vi "Matlab Chirps Computation.vi"(7 "Movement correction":bool, 8 "error in":errorcluster, 9 "Zoom":dbl[](array[numeric]), 10 "ROI Coordinates":T3={"XYZ Start"=[{"X"=-1.0, "Y"=-1.0, "Z"=0.0}, {"X"=-1.0, "Y"=-0.99, "Z"=0.0}, {"X"=-1.0, "Y"=-0.98, "Z"=0.0}, {"X"=-1.0, "Y"=-0.97, "Z"=0.0}, {"X"=-1.0, "Y"=-0.96, "Z"=0.0}, {"X"=-1.0, "Y"=-0.95, "Z"=0.0}, {"X"=-1.0, "Y"=-0.94, "Z"=0.0}, {"X"=-1.0, "Y"=-0.93, "Z"=0.0}, {"X"=-1.0, "Y"=-0.92, "Z"=0.0}, {"X"=-1.0, "Y"=-0.91, "Z"=0.0}, {"X"=-1.0, "Y"=-0.9, "Z"=0.0}, {"X"=-1.0, "Y"=-0.89, "Z"=0.0}, {"X"=-1.0, "Y"=-0.88, "Z"=0.0}, {"X"=-1.0, "Y"=-0.87, "Z"=0.0}, {"X"=-1.0, "Y"=-0.86, "Z"=0.0}, {"X"=-1.0, "Y"=-0.85, "Z"=0.0}, {"X"=-1.0, "Y"=-0.84, "Z"=0.0}, {"X"=-1.0, "Y"=-0.83, "Z"=0.0}, {"X"=-1.0, "Y"=-0.82, "Z"=0.0}, {"X"=-1.0, "Y"=-0.81, "Z"=0.0}, {"X"=-1.0, "Y"=-0.8, "Z"=0.0}, {"X"=-1.0, "Y"=-0.79, "Z"=0.0}, {"X"=-1.0, "Y"=-0.78, "Z"=0.0}, {"X"=-1.0, "Y"=-0.77, "Z"=0.0}, {"X"=-1.0, "Y"=-0.76, "Z"=0.0}, {"X"=-1.0, "Y"=-0.75, "Z"=0.0}, {"X"=-1.0, "Y"=-0.74, "Z"=0.0}, {"X"=-1.0, "Y"=-0.73, "Z"=0.0}, {"X"=-1.0, "Y"=-0.72, "Z"=0.0}, {"X"=-1.0, "Y"=-0.71, "Z"=0.0}, {"X"=-1.0, "Y"=-0.7, "Z"=0.0}, {"X"=-1.0, "Y"=-0.69, "Z"=0.0}, {"X"=-1.0, "Y"=-0.68, "Z"=0.0}, {"X"=-1.0, "Y"=-0.67, "Z"=0.0}, {"X"=-1.0, "Y"=-0.66, "Z"=0.0}, {"X"=-1.0, "Y"=-0.65, "Z"=0.0}, {"X"=-1.0, "Y"=-0.64, "Z"=0.0}, {"X"=-1.0, "Y"=-0.63, "Z"=0.0}, {"X"=-1.0, "Y"=-0.62, "Z"=0.0}, {"X"=-1.0, "Y"=-0.61, "Z"=0.0}, {"X"=-1.0, "Y"=-0.6, "Z"=0.0}, {"X"=-1.0, "Y"=-0.59, "Z"=0.0}, {"X"=-1.0, "Y"=-0.58, "Z"=0.0}, {"X"=-1.0, "Y"=-0.57, "Z"=0.0}, {"X"=-1.0, "Y"=-0.56, "Z"=0.0}, {"X"=-1.0, "Y"=-0.55, "Z"=0.0}, {"X"=-1.0, "Y"=-0.54, "Z"=0.0}, {"X"=-1.0, "Y"=-0.53, "Z"=0.0}, {"X"=-1.0, "Y"=-0.52, "Z"=0.0}, {"X"=-1.0, "Y"=-0.51, "Z"=0.0}, {"X"=-1.0, "Y"=-0.5, "Z"=0.0}, {"X"=-1.0, "Y"=-0.49, "Z"=0.0}, {"X"=-1.0, "Y"=-0.48, "Z"=0.0}, {"X"=-1.0, "Y"=-0.47, "Z"=0.0}, {"X"=-1.0, "Y"=-0.46, "Z"=0.0}, {"X"=-1.0, "Y"=-0.45, "Z"=0.0}, {"X"=-1.0, "Y"=-0.44, "Z"=0.0}, {"X"=-1.0, "Y"=-0.43, "Z"=0.0}, {"X"=-1.0, "Y"=-0.42, "Z"=0.0}, {"X"=-1.0, "Y"=-0.41, "Z"=0.0}, {"X"=-1.0, "Y"=-0.4, "Z"=0.0}, {"X"=-1.0, "Y"=-0.39, "Z"=0.0}, {"X"=-1.0, "Y"=-0.38, "Z"=0.0}, {"X"=-1.0, "Y"=-0.37, "Z"=0.0}, {"X"=-1.0, "Y"=-0.36, "Z"=0.0}, {"X"=-1.0, "Y"=-0.35, "Z"=0.0}, {"X"=-1.0, "Y"=-0.34, "Z"=0.0}, {"X"=-1.0, "Y"=-0.33, "Z"=0.0}, {"X"=-1.0, "Y"=-0.32, "Z"=0.0}, {"X"=-1.0, "Y"=-0.31, "Z"=0.0}, {"X"=-1.0, "Y"=-0.3, "Z"=0.0}, {"X"=-1.0, "Y"=-0.29, "Z"=0.0}, {"X"=-1.0, "Y"=-0.28, "Z"=0.0}, {"X"=-1.0, "Y"=-0.27, "Z"=0.0}, {"X"=-1.0, "Y"=-0.26, "Z"=0.0}, {"X"=-1.0, "Y"=-0.25, "Z"=0.0}, {"X"=-1.0, "Y"=-0.24, "Z"=0.0}, {"X"=-1.0, "Y"=-0.23, "Z"=0.0}, {"X"=-1.0, "Y"=-0.22, "Z"=0.0}, {"X"=-1.0, "Y"=-0.21, "Z"=0.0}, {"X"=-1.0, "Y"=-0.2, "Z"=0.0}, {"X"=-1.0, "Y"=-0.19, "Z"=0.0}, {"X"=-1.0, "Y"=-0.18, "Z"=0.0}, {"X"=-1.0, "Y"=-0.17, "Z"=0.0}, {"X"=-1.0, "Y"=-0.16, "Z"=0.0}, {"X"=-1.0, "Y"=-0.15, "Z"=0.0}, {"X"=-1.0, "Y"=-0.14, "Z"=0.0}, {"X"=-1.0, "Y"=-0.13, "Z"=0.0}, {"X"=-1.0, "Y"=-0.12, "Z"=0.0}, {"X"=-1.0, "Y"=-0.11, "Z"=0.0}, {"X"=-1.0, "Y"=-0.1, "Z"=0.0}, {"X"=-1.0, "Y"=-0.09, "Z"=0.0}, {"X"=-1.0, "Y"=-0.08, "Z"=0.0}, {"X"=-1.0, "Y"=-0.07, "Z"=0.0}, {"X"=-1.0, "Y"=-0.06, "Z"=0.0}, {"X"=-1.0, "Y"=-0.05, "Z"=0.0}, {"X"=-1.0, "Y"=-0.04, "Z"=0.0}, {"X"=-1.0, "Y"=-0.03, "Z"=0.0}, {"X"=-1.0, "Y"=-0.02, "Z"=0.0}, {"X"=-1.0, "Y"=-0.01, "Z"=0.0}, {"X"=-1.0, "Y"=0.0, "Z"=0.0}, {"X"=-1.0, "Y"=0.01, "Z"=0.0}, {"X"=-1.0, "Y"=0.02, "Z"=0.0}, {"X"=-1.0, "Y"=0.03, "Z"=0.0}, {"X"=-1.0, "Y"=0.04, "Z"=0.0}, {"X"=-1.0, "Y"=0.05, "Z"=0.0}, {"X"=-1.0, "Y"=0.06, "Z"=0.0}, {"X"=-1.0, "Y"=0.07, "Z"=0.0}, {"X"=-1.0, "Y"=0.08, "Z"=0.0}, {"X"=-1.0, "Y"=0.09, "Z"=0.0}, {"X"=-1.0, "Y"=0.1, "Z"=0.0}, {"X"=-1.0, "Y"=0.11, "Z"=0.0}, {"X"=-1.0, "Y"=0.12, "Z"=0.0}, {"X"=-1.0, "Y"=0.13, "Z"=0.0}, {"X"=-1.0, "Y"=0.14, "Z"=0.0}, {"X"=-1.0, "Y"=0.15, "Z"=0.0}, {"X"=-1.0, "Y"=0.16, "Z"=0.0}, {"X"=-1.0, "Y"=0.17, "Z"=0.0}, {"X"=-1.0, "Y"=0.18, "Z"=0.0}, {"X"=-1.0, "Y"=0.19, "Z"=0.0}, {"X"=-1.0, "Y"=0.2, "Z"=0.0}, {"X"=-1.0, "Y"=0.21, "Z"=0.0}, {"X"=-1.0, "Y"=0.22, "Z"=0.0}, {"X"=-1.0, "Y"=0.23, "Z"=0.0}, {"X"=-1.0, "Y"=0.24, "Z"=0.0}, {"X"=-1.0, "Y"=0.25, "Z"=0.0}, {"X"=-1.0, "Y"=0.26, "Z"=0.0}, {"X"=-1.0, "Y"=0.27, "Z"=0.0}, {"X"=-1.0, "Y"=0.28, "Z"=0.0}, {"X"=-1.0, "Y"=0.29, "Z"=0.0}, {"X"=-1.0, "Y"=0.3, "Z"=0.0}, {"X"=-1.0, "Y"=0.31, "Z"=0.0}, {"X"=-1.0, "Y"=0.32, "Z"=0.0}, {"X"=-1.0, "Y"=0.33, "Z"=0.0}, {"X"=-1.0, "Y"=0.34, "Z"=0.0}, {"X"=-1.0, "Y"=0.35, "Z"=0.0}, {"X"=-1.0, "Y"=0.36, "Z"=0.0}, {"X"=-1.0, "Y"=0.37, "Z"=0.0}, {"X"=-1.0, "Y"=0.38, "Z"=0.0}, {"X"=-1.0, "Y"=0.39, "Z"=0.0}, {"X"=-1.0, "Y"=0.4, "Z"=0.0}, {"X"=-1.0, "Y"=0.41, "Z"=0.0}, {"X"=-1.0, "Y"=0.42, "Z"=0.0}, {"X"=-1.0, "Y"=0.43, "Z"=0.0}, {"X"=-1.0, "Y"=0.44, "Z"=0.0}, {"X"=-1.0, "Y"=0.45, "Z"=0.0}, {"X"=-1.0, "Y"=0.46, "Z"=0.0}, {"X"=-1.0, "Y"=0.47, "Z"=0.0}, {"X"=-1.0, "Y"=0.48, "Z"=0.0}, {"X"=-1.0, "Y"=0.49, "Z"=0.0}, {"X"=-1.0, "Y"=0.5, "Z"=0.0}, {"X"=-1.0, "Y"=0.51, "Z"=0.0}, {"X"=-1.0, "Y"=0.52, "Z"=0.0}, {"X"=-1.0, "Y"=0.53, "Z"=0.0}, {"X"=-1.0, "Y"=0.54, "Z"=0.0}, {"X"=-1.0, "Y"=0.55, "Z"=0.0}, {"X"=-1.0, "Y"=0.56, "Z"=0.0}, {"X"=-1.0, "Y"=0.57, "Z"=0.0}, {"X"=-1.0, "Y"=0.58, "Z"=0.0}, {"X"=-1.0, "Y"=0.59, "Z"=0.0}, {"X"=-1.0, "Y"=0.6, "Z"=0.0}, {"X"=-1.0, "Y"=0.61, "Z"=0.0}, {"X"=-1.0, "Y"=0.62, "Z"=0.0}, {"X"=-1.0, "Y"=0.63, "Z"=0.0}, {"X"=-1.0, "Y"=0.64, "Z"=0.0}, {"X"=-1.0, "Y"=0.65, "Z"=0.0}, {"X"=-1.0, "Y"=0.66, "Z"=0.0}, {"X"=-1.0, "Y"=0.67, "Z"=0.0}, {"X"=-1.0, "Y"=0.68, "Z"=0.0}, {"X"=-1.0, "Y"=0.69, "Z"=0.0}, {"X"=-1.0, "Y"=0.7, "Z"=0.0}, {"X"=-1.0, "Y"=0.71, "Z"=0.0}, {"X"=-1.0, "Y"=0.72, "Z"=0.0}, {"X"=-1.0, "Y"=0.73, "Z"=0.0}, {"X"=-1.0, "Y"=0.74, "Z"=0.0}, {"X"=-1.0, "Y"=0.75, "Z"=0.0}, {"X"=-1.0, "Y"=0.76, "Z"=0.0}, {"X"=-1.0, "Y"=0.77, "Z"=0.0}, {"X"=-1.0, "Y"=0.78, "Z"=0.0}, {"X"=-1.0, "Y"=0.79, "Z"=0.0}, {"X"=-1.0, "Y"=0.8, "Z"=0.0}, {"X"=-1.0, "Y"=0.81, "Z"=0.0}, {"X"=-1.0, "Y"=0.82, "Z"=0.0}, {"X"=-1.0, "Y"=0.83, "Z"=0.0}, {"X"=-1.0, "Y"=0.84, "Z"=0.0}, {"X"=-1.0, "Y"=0.85, "Z"=0.0}, {"X"=-1.0, "Y"=0.86, "Z"=0.0}, {"X"=-1.0, "Y"=0.87, "Z"=0.0}, {"X"=-1.0, "Y"=0.88, "Z"=0.0}, {"X"=-1.0, "Y"=0.89, "Z"=0.0}, {"X"=-1.0, "Y"=0.9, "Z"=0.0}, {"X"=-1.0, "Y"=0.91, "Z"=0.0}, {"X"=-1.0, "Y"=0.92, "Z"=0.0}, {"X"=-1.0, "Y"=0.93, "Z"=0.0}, {"X"=-1.0, "Y"=0.94, "Z"=0.0}, {"X"=-1.0, "Y"=0.95, "Z"=0.0}, {"X"=-1.0, "Y"=0.96, "Z"=0.0}, {"X"=-1.0, "Y"=0.97, "Z"=0.0}, {"X"=-1.0, "Y"=0.98, "Z"=0.0}, {"X"=-1.0, "Y"=0.99, "Z"=0.0}], "XYZ Stop"=[{"X"=1.0, "Y"=-1.0, "Z"=0.0}, {"X"=1.0, "Y"=-0.99, "Z"=0.0}, {"X"=1.0, "Y"=-0.98, "Z"=0.0}, {"X"=1.0, "Y"=-0.97, "Z"=0.0}, {"X"=1.0, "Y"=-0.96, "Z"=0.0}, {"X"=1.0, "Y"=-0.95, "Z"=0.0}, {"X"=1.0, "Y"=-0.94, "Z"=0.0}, {"X"=1.0, "Y"=-0.93, "Z"=0.0}, {"X"=1.0, "Y"=-0.92, "Z"=0.0}, {"X"=1.0, "Y"=-0.91, "Z"=0.0}, {"X"=1.0, "Y"=-0.9, "Z"=0.0}, {"X"=1.0, "Y"=-0.89, "Z"=0.0}, {"X"=1.0, "Y"=-0.88, "Z"=0.0}, {"X"=1.0, "Y"=-0.87, "Z"=0.0}, {"X"=1.0, "Y"=-0.86, "Z"=0.0}, {"X"=1.0, "Y"=-0.85, "Z"=0.0}, {"X"=1.0, "Y"=-0.84, "Z"=0.0}, {"X"=1.0, "Y"=-0.83, "Z"=0.0}, {"X"=1.0, "Y"=-0.82, "Z"=0.0}, {"X"=1.0, "Y"=-0.81, "Z"=0.0}, {"X"=1.0, "Y"=-0.8, "Z"=0.0}, {"X"=1.0, "Y"=-0.79, "Z"=0.0}, {"X"=1.0, "Y"=-0.78, "Z"=0.0}, {"X"=1.0, "Y"=-0.77, "Z"=0.0}, {"X"=1.0, "Y"=-0.76, "Z"=0.0}, {"X"=1.0, "Y"=-0.75, "Z"=0.0}, {"X"=1.0, "Y"=-0.74, "Z"=0.0}, {"X"=1.0, "Y"=-0.73, "Z"=0.0}, {"X"=1.0, "Y"=-0.72, "Z"=0.0}, {"X"=1.0, "Y"=-0.71, "Z"=0.0}, {"X"=1.0, "Y"=-0.7, "Z"=0.0}, {"X"=1.0, "Y"=-0.69, "Z"=0.0}, {"X"=1.0, "Y"=-0.68, "Z"=0.0}, {"X"=1.0, "Y"=-0.67, "Z"=0.0}, {"X"=1.0, "Y"=-0.66, "Z"=0.0}, {"X"=1.0, "Y"=-0.65, "Z"=0.0}, {"X"=1.0, "Y"=-0.64, "Z"=0.0}, {"X"=1.0, "Y"=-0.63, "Z"=0.0}, {"X"=1.0, "Y"=-0.62, "Z"=0.0}, {"X"=1.0, "Y"=-0.61, "Z"=0.0}, {"X"=1.0, "Y"=-0.6, "Z"=0.0}, {"X"=1.0, "Y"=-0.59, "Z"=0.0}, {"X"=1.0, "Y"=-0.58, "Z"=0.0}, {"X"=1.0, "Y"=-0.57, "Z"=0.0}, {"X"=1.0, "Y"=-0.56, "Z"=0.0}, {"X"=1.0, "Y"=-0.55, "Z"=0.0}, {"X"=1.0, "Y"=-0.54, "Z"=0.0}, {"X"=1.0, "Y"=-0.53, "Z"=0.0}, {"X"=1.0, "Y"=-0.52, "Z"=0.0}, {"X"=1.0, "Y"=-0.51, "Z"=0.0}, {"X"=1.0, "Y"=-0.5, "Z"=0.0}, {"X"=1.0, "Y"=-0.49, "Z"=0.0}, {"X"=1.0, "Y"=-0.48, "Z"=0.0}, {"X"=1.0, "Y"=-0.47, "Z"=0.0}, {"X"=1.0, "Y"=-0.46, "Z"=0.0}, {"X"=1.0, "Y"=-0.45, "Z"=0.0}, {"X"=1.0, "Y"=-0.44, "Z"=0.0}, {"X"=1.0, "Y"=-0.43, "Z"=0.0}, {"X"=1.0, "Y"=-0.42, "Z"=0.0}, {"X"=1.0, "Y"=-0.41, "Z"=0.0}, {"X"=1.0, "Y"=-0.4, "Z"=0.0}, {"X"=1.0, "Y"=-0.39, "Z"=0.0}, {"X"=1.0, "Y"=-0.38, "Z"=0.0}, {"X"=1.0, "Y"=-0.37, "Z"=0.0}, {"X"=1.0, "Y"=-0.36, "Z"=0.0}, {"X"=1.0, "Y"=-0.35, "Z"=0.0}, {"X"=1.0, "Y"=-0.34, "Z"=0.0}, {"X"=1.0, "Y"=-0.33, "Z"=0.0}, {"X"=1.0, "Y"=-0.32, "Z"=0.0}, {"X"=1.0, "Y"=-0.31, "Z"=0.0}, {"X"=1.0, "Y"=-0.3, "Z"=0.0}, {"X"=1.0, "Y"=-0.29, "Z"=0.0}, {"X"=1.0, "Y"=-0.28, "Z"=0.0}, {"X"=1.0, "Y"=-0.27, "Z"=0.0}, {"X"=1.0, "Y"=-0.26, "Z"=0.0}, {"X"=1.0, "Y"=-0.25, "Z"=0.0}, {"X"=1.0, "Y"=-0.24, "Z"=0.0}, {"X"=1.0, "Y"=-0.23, "Z"=0.0}, {"X"=1.0, "Y"=-0.22, "Z"=0.0}, {"X"=1.0, "Y"=-0.21, "Z"=0.0}, {"X"=1.0, "Y"=-0.2, "Z"=0.0}, {"X"=1.0, "Y"=-0.19, "Z"=0.0}, {"X"=1.0, "Y"=-0.18, "Z"=0.0}, {"X"=1.0, "Y"=-0.17, "Z"=0.0}, {"X"=1.0, "Y"=-0.16, "Z"=0.0}, {"X"=1.0, "Y"=-0.15, "Z"=0.0}, {"X"=1.0, "Y"=-0.14, "Z"=0.0}, {"X"=1.0, "Y"=-0.13, "Z"=0.0}, {"X"=1.0, "Y"=-0.12, "Z"=0.0}, {"X"=1.0, "Y"=-0.11, "Z"=0.0}, {"X"=1.0, "Y"=-0.1, "Z"=0.0}, {"X"=1.0, "Y"=-0.09, "Z"=0.0}, {"X"=1.0, "Y"=-0.08, "Z"=0.0}, {"X"=1.0, "Y"=-0.07, "Z"=0.0}, {"X"=1.0, "Y"=-0.06, "Z"=0.0}, {"X"=1.0, "Y"=-0.05, "Z"=0.0}, {"X"=1.0, "Y"=-0.04, "Z"=0.0}, {"X"=1.0, "Y"=-0.03, "Z"=0.0}, {"X"=1.0, "Y"=-0.02, "Z"=0.0}, {"X"=1.0, "Y"=-0.01, "Z"=0.0}, {"X"=1.0, "Y"=0.0, "Z"=0.0}, {"X"=1.0, "Y"=0.01, "Z"=0.0}, {"X"=1.0, "Y"=0.02, "Z"=0.0}, {"X"=1.0, "Y"=0.03, "Z"=0.0}, {"X"=1.0, "Y"=0.04, "Z"=0.0}, {"X"=1.0, "Y"=0.05, "Z"=0.0}, {"X"=1.0, "Y"=0.06, "Z"=0.0}, {"X"=1.0, "Y"=0.07, "Z"=0.0}, {"X"=1.0, "Y"=0.08, "Z"=0.0}, {"X"=1.0, "Y"=0.09, "Z"=0.0}, {"X"=1.0, "Y"=0.1, "Z"=0.0}, {"X"=1.0, "Y"=0.11, "Z"=0.0}, {"X"=1.0, "Y"=0.12, "Z"=0.0}, {"X"=1.0, "Y"=0.13, "Z"=0.0}, {"X"=1.0, "Y"=0.14, "Z"=0.0}, {"X"=1.0, "Y"=0.15, "Z"=0.0}, {"X"=1.0, "Y"=0.16, "Z"=0.0}, {"X"=1.0, "Y"=0.17, "Z"=0.0}, {"X"=1.0, "Y"=0.18, "Z"=0.0}, {"X"=1.0, "Y"=0.19, "Z"=0.0}, {"X"=1.0, "Y"=0.2, "Z"=0.0}, {"X"=1.0, "Y"=0.21, "Z"=0.0}, {"X"=1.0, "Y"=0.22, "Z"=0.0}, {"X"=1.0, "Y"=0.23, "Z"=0.0}, {"X"=1.0, "Y"=0.24, "Z"=0.0}, {"X"=1.0, "Y"=0.25, "Z"=0.0}, {"X"=1.0, "Y"=0.26, "Z"=0.0}, {"X"=1.0, "Y"=0.27, "Z"=0.0}, {"X"=1.0, "Y"=0.28, "Z"=0.0}, {"X"=1.0, "Y"=0.29, "Z"=0.0}, {"X"=1.0, "Y"=0.3, "Z"=0.0}, {"X"=1.0, "Y"=0.31, "Z"=0.0}, {"X"=1.0, "Y"=0.32, "Z"=0.0}, {"X"=1.0, "Y"=0.33, "Z"=0.0}, {"X"=1.0, "Y"=0.34, "Z"=0.0}, {"X"=1.0, "Y"=0.35, "Z"=0.0}, {"X"=1.0, "Y"=0.36, "Z"=0.0}, {"X"=1.0, "Y"=0.37, "Z"=0.0}, {"X"=1.0, "Y"=0.38, "Z"=0.0}, {"X"=1.0, "Y"=0.39, "Z"=0.0}, {"X"=1.0, "Y"=0.4, "Z"=0.0}, {"X"=1.0, "Y"=0.41, "Z"=0.0}, {"X"=1.0, "Y"=0.42, "Z"=0.0}, {"X"=1.0, "Y"=0.43, "Z"=0.0}, {"X"=1.0, "Y"=0.44, "Z"=0.0}, {"X"=1.0, "Y"=0.45, "Z"=0.0}, {"X"=1.0, "Y"=0.46, "Z"=0.0}, {"X"=1.0, "Y"=0.47, "Z"=0.0}, {"X"=1.0, "Y"=0.48, "Z"=0.0}, {"X"=1.0, "Y"=0.49, "Z"=0.0}, {"X"=1.0, "Y"=0.5, "Z"=0.0}, {"X"=1.0, "Y"=0.51, "Z"=0.0}, {"X"=1.0, "Y"=0.52, "Z"=0.0}, {"X"=1.0, "Y"=0.53, "Z"=0.0}, {"X"=1.0, "Y"=0.54, "Z"=0.0}, {"X"=1.0, "Y"=0.55, "Z"=0.0}, {"X"=1.0, "Y"=0.56, "Z"=0.0}, {"X"=1.0, "Y"=0.57, "Z"=0.0}, {"X"=1.0, "Y"=0.58, "Z"=0.0}, {"X"=1.0, "Y"=0.59, "Z"=0.0}, {"X"=1.0, "Y"=0.6, "Z"=0.0}, {"X"=1.0, "Y"=0.61, "Z"=0.0}, {"X"=1.0, "Y"=0.62, "Z"=0.0}, {"X"=1.0, "Y"=0.63, "Z"=0.0}, {"X"=1.0, "Y"=0.64, "Z"=0.0}, {"X"=1.0, "Y"=0.65, "Z"=0.0}, {"X"=1.0, "Y"=0.66, "Z"=0.0}, {"X"=1.0, "Y"=0.67, "Z"=0.0}, {"X"=1.0, "Y"=0.68, "Z"=0.0}, {"X"=1.0, "Y"=0.69, "Z"=0.0}, {"X"=1.0, "Y"=0.7, "Z"=0.0}, {"X"=1.0, "Y"=0.71, "Z"=0.0}, {"X"=1.0, "Y"=0.72, "Z"=0.0}, {"X"=1.0, "Y"=0.73, "Z"=0.0}, {"X"=1.0, "Y"=0.74, "Z"=0.0}, {"X"=1.0, "Y"=0.75, "Z"=0.0}, {"X"=1.0, "Y"=0.76, "Z"=0.0}, {"X"=1.0, "Y"=0.77, "Z"=0.0}, {"X"=1.0, "Y"=0.78, "Z"=0.0}, {"X"=1.0, "Y"=0.79, "Z"=0.0}, {"X"=1.0, "Y"=0.8, "Z"=0.0}, {"X"=1.0, "Y"=0.81, "Z"=0.0}, {"X"=1.0, "Y"=0.82, "Z"=0.0}, {"X"=1.0, "Y"=0.83, "Z"=0.0}, {"X"=1.0, "Y"=0.84, "Z"=0.0}, {"X"=1.0, "Y"=0.85, "Z"=0.0}, {"X"=1.0, "Y"=0.86, "Z"=0.0}, {"X"=1.0, "Y"=0.87, "Z"=0.0}, {"X"=1.0, "Y"=0.88, "Z"=0.0}, {"X"=1.0, "Y"=0.89, "Z"=0.0}, {"X"=1.0, "Y"=0.9, "Z"=0.0}, {"X"=1.0, "Y"=0.91, "Z"=0.0}, {"X"=1.0, "Y"=0.92, "Z"=0.0}, {"X"=1.0, "Y"=0.93, "Z"=0.0}, {"X"=1.0, "Y"=0.94, "Z"=0.0}, {"X"=1.0, "Y"=0.95, "Z"=0.0}, {"X"=1.0, "Y"=0.96, "Z"=0.0}, {"X"=1.0, "Y"=0.97, "Z"=0.0}, {"X"=1.0, "Y"=0.98, "Z"=0.0}, {"X"=1.0, "Y"=0.99, "Z"=0.0}]}, 11 "AOL_Globals":T4={"Imaging Protocol"=enum."Live Imaging", "Number of POI"=0, "Number of Miniscans"=0, "Number of Trials"=1, "Number of Cycles "=0, "# Averaged Frames"=1, "Laser power (%)"=7, "Pockels (V)"=0.0, "Acquisition Length (sec)"=0.0, "Fill time (us)"=24.5, "POI Dwell time (us)"=4.0, "Miniscan Dwell time per pixel (us)"=0.0, "PMT 1"=500.0, "PMT 2"=500.0, "Back Apperture (mA)"=0.0, "Frame Size"=200, "Center Frequency"=36.28048780487805, "Field of View (um)"=175.0, "Field of View (norm)"=4.349999904632568, "DwellTime (us)"=0.1, "Ref Dwell Time (us)"=0.0, "Wavelength (nm)"=820.0, "Zoom"=1.0, "AOL Z"=0.0, "AOL Mode"=enum."Raster", "GridXY"=0.0, "GridZ"=0.0, "TriggerPeriod (sec)"=0.0, "Number of Pixels in Miniscan"=0, "Experiment folder path"=path "", "X centre"=0.0, "Y centre"=0.0, "Angle (degrees)"=0.0, "Angle Xs (degrees)"=0.0, "Angle Ys (degrees)"=0.0, "Plane Mode"=0, "Threshold"=[], "Regenerate Chirps"=FALSE, "Rectangle ROI length (pixels)"=0, "Rectangle ROI height (pixels)"=0, "AOD fill"=4900, "StartupDelay"=0, "Samples Wait after Trigger"=5080, "Slip Cycle"=600000, "Add Cycle"=TRUE, "Functional Mode"=enum."Point", "Z Start"=0.0, "Z Stop"=0.0, "# Planes"=0, "Total Pixels"=0, "Variable Miniscan Pixels"=[], "Use Variable Length"=FALSE, "Use Variable Resolution"=FALSE, "Laser power (%) at Z Start"=0, "Laser power (%) at Z Stop"=0, "Ref Z Step"=0} {"Angle Ys (degrees)" format="%#.6g"; "Angle Xs (degrees)" format="%#.6g"; "Plane Mode" items=["XY Plane", "XZ Plane", "YZ Plane", "arbitraryplane"]; "Frame Size" items=["100X100"=100, "128X128"=128, "200X200"=200, "256X256"=256, "512X512"=512, "1024x1024"=1024, "2048x2048"=2048]; "Back Apperture (mA)" format="%#.6g"; "Pockels (V)" format="%#.6g"; "PMT 2" format="%#.6g"; "PMT 1" format="%#.6g"; "Angle (degrees)" format="%#.6g"; "POI Dwell time (us)" format="%#.6g"}) -> (0 "error out":errorcluster, 2 "scanVariables":dbl[][](array[numeric]), 3 "Chirp Parameters":T2, 4 "Execution time (ms)":u32)   [LabVIEW 2020]
uses:
  Typedefs/Controls/AOL_Globals.ctl
  Typedefs/Imaging Protocols enum.ctl
  Typedefs/Frame Size.ctl
  Typedefs/AOL modes.ctl
  Typedefs/Plane Mode.ctl
  Typedefs/Functional Mode.ctl
  Typedefs/Chirp_ABCD.ctl
panel:
  in  "Stantalone {F} ?":bool
  in  "Tab Control":T1(tab)
  out "XYZ Array size":i32[](array[numeric])
  out "Use Variable Length":bool
  out "Number of Miniscans":u16
  out "Chirp Array size":i32[](array[numeric])
  out "Pixels per miniscan":dbl[](array[numeric])
  out "D":dbl[][](array[numeric])
  out "C":dbl[][](array[numeric])
  out "B":dbl[][](array[numeric])
  out "A":dbl[][](array[numeric])
  out "t":dbl[][](array[numeric])
  out "Timing_offsets":dbl[][](array[numeric])
  out "Distortion corr":dbl
  out "delta_bz":dbl[][](array[numeric]) format="%#.6g"
  out "delta_a_dz":dbl[][](array[numeric])
  out "d_4app":dbl[][](array[numeric])
  out "timings_offsets":dbl[](array[numeric])
  out "T_ramp All":dbl[][](graph)
  out "T_ramp Intensity Graph":dbl[][](graph)
  out "A  All":dbl[][](graph)
  out "A Intensity Graph 2":dbl[][](graph)
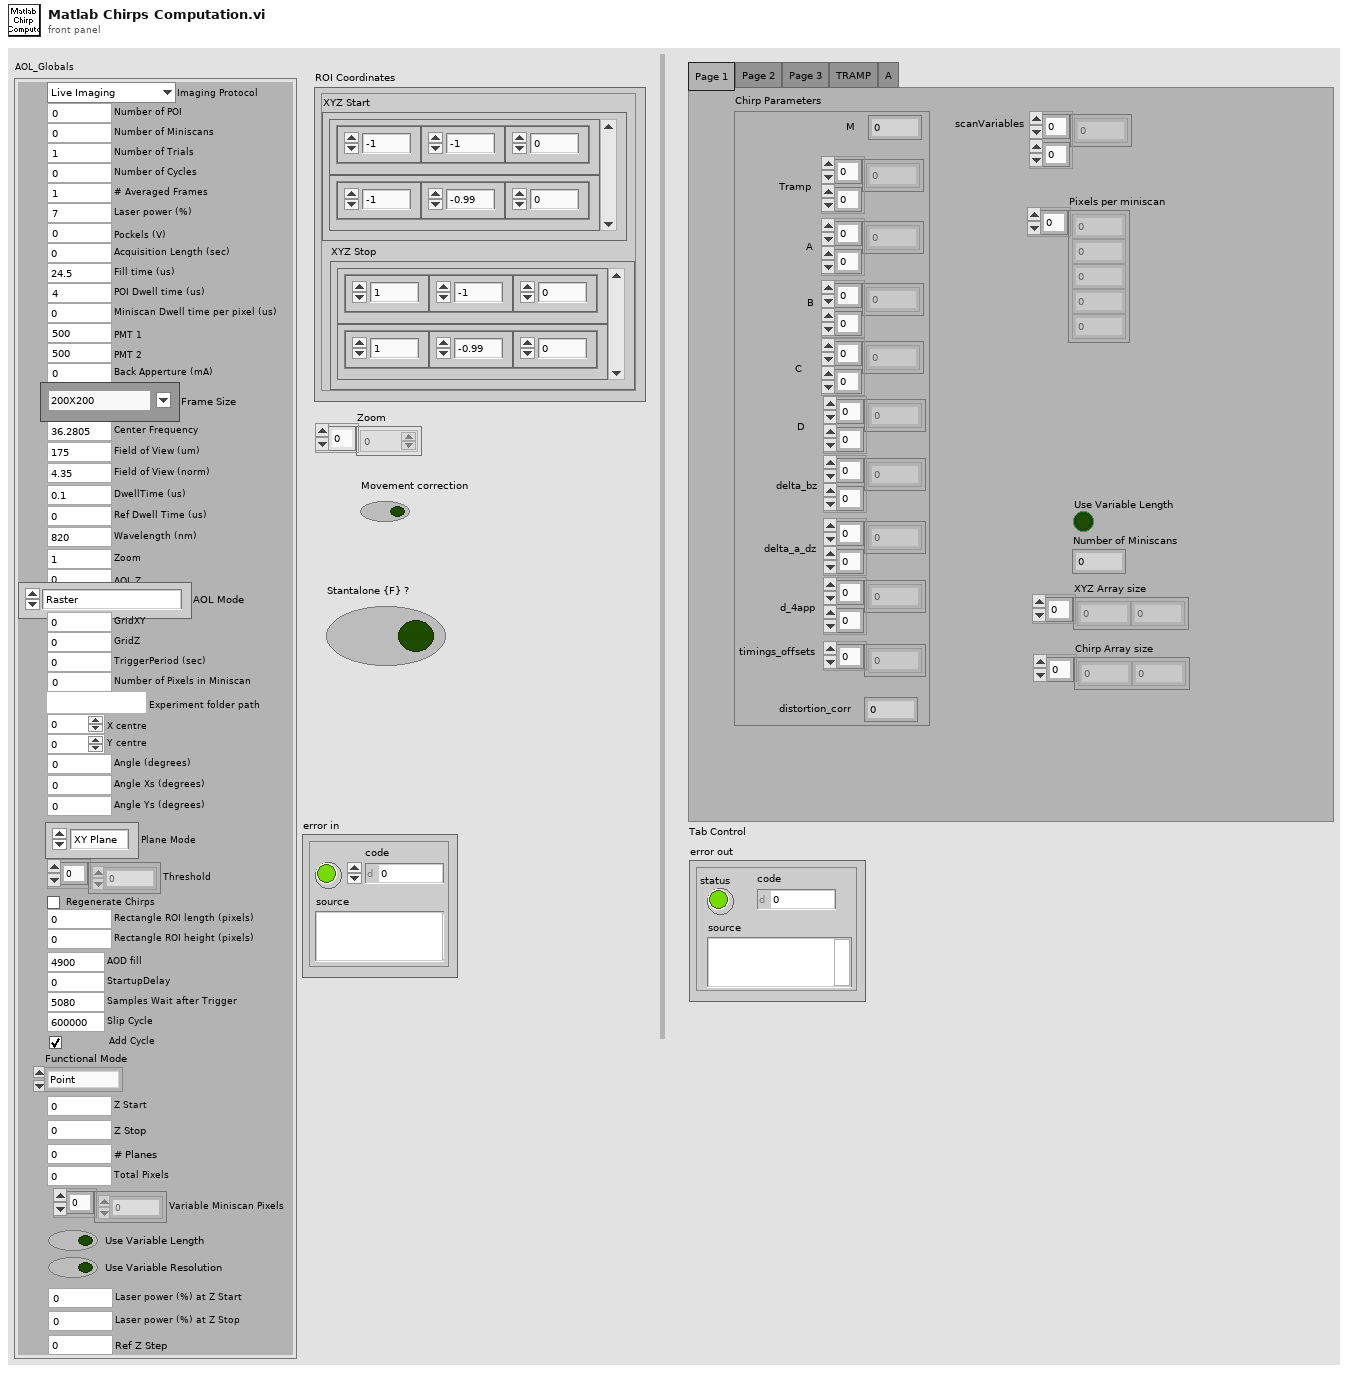
[diagram p1: front panel]
types:
  T1 = enum32{"Page 1", "Page 2", "Page 3", "TRAMP", "A"}
  T2 = typedef "Chirp_ABCD.ctl" = cluster{"M ":dbl, "Tramp":dbl[][], "A":dbl[][], "B":dbl[][], "C":dbl[][], "D":dbl[][], "delta_bz":dbl[][], "delta_a_dz":dbl[][], "d_4app":dbl[][], "timings_offsets":dbl[], "distortion_corr":dbl}
  T3 = cluster{"XYZ Start":cluster{"X":sgl, "Y":sgl, "Z":sgl}[], "XYZ Stop":cluster{"X":sgl, "Y":sgl, "Z":sgl}[]}
  T4 = typedef "AOL_Globals.ctl" = cluster{"Imaging Protocol":T5, "Number of POI":u16, "Number of Miniscans":u16, "Number of Trials":u16, "Number of Cycles ":u64, "# Averaged Frames":u16, "Laser power (%)":u8, "Pockels (V)":dbl, "Acquisition Length (sec)":dbl, "Fill time (us)":dbl, "POI Dwell time (us)":dbl, "Miniscan Dwell time per pixel (us)":dbl, "PMT 1":dbl, "PMT 2":dbl, "Back Apperture (mA)":dbl, "Frame Size":T6, "Center Frequency":dbl, "Field of View (um)":dbl, "Field of View (norm)":dbl, "DwellTime (us)":dbl, "Ref Dwell Time (us)":dbl, "Wavelength (nm)":dbl, "Zoom":dbl, "AOL Z":dbl, "AOL Mode":T7, "GridXY":dbl, "GridZ":dbl, "TriggerPeriod (sec)":dbl, "Number of Pixels in Miniscan":u16, "Experiment folder path":path, "X centre":dbl, "Y centre":dbl, "Angle (degrees)":dbl, "Angle Xs (degrees)":dbl, "Angle Ys (degrees)":dbl, "Plane Mode":T8, "Threshold":u16[], "Regenerate Chirps":bool, "Rectangle ROI length (pixels)":u16, "Rectangle ROI height (pixels)":u16, "AOD fill":u16, "StartupDelay":i32, "Samples Wait after Trigger":u16, "Slip Cycle":u32, "Add Cycle":bool, "Functional Mode":T9, "Z Start":dbl, "Z Stop":dbl, "# Planes":i32, "Total Pixels":i32, "Variable Miniscan Pixels":u16[], "Use Variable Length":bool, "Use Variable Resolution":bool, "Laser power (%) at Z Start":u8, "Laser power (%) at Z Stop":u8, "Ref Z Step":i8}
  T5 = typedef "Imaging Protocols enum.ctl" = enum16{"AOL Z-Stack", "Motor Z Stack", "Parameter Sweep", "Functional Acquisition", "Single Plane Acquisition", "Volume Acquisition", "Live Imaging", "Live Plane Imaging", "Live Volume Imaging"}
  T6 = typedef "Frame Size.ctl" = u16
  T7 = typedef "AOL modes.ctl" = enum16{"Raster", "Structural", "Pointing", "Mini Scan", "Alignment"}
  T8 = typedef "Plane Mode.ctl" = u16
  T9 = typedef "Functional Mode.ctl" = enum16{"Point", "Line", "Patch", "Plane", "Volume"}
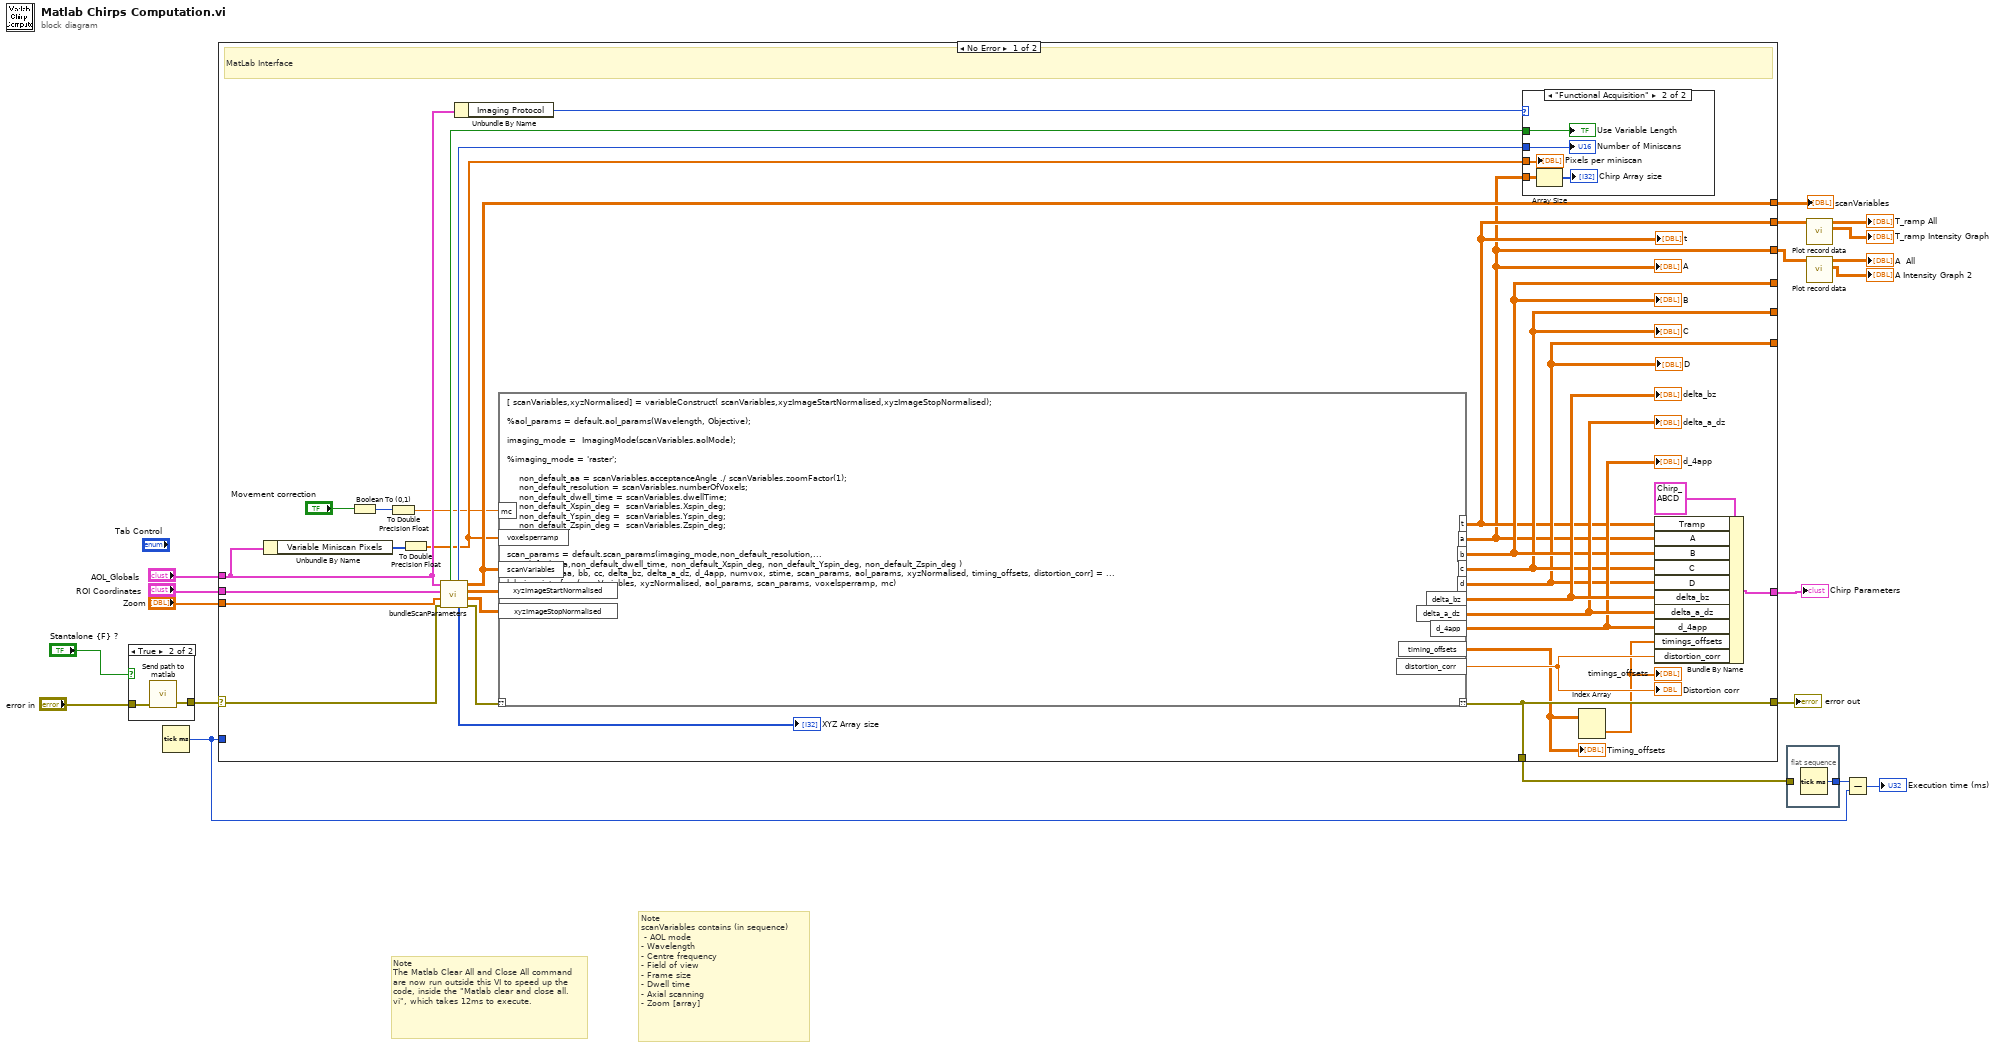
[diagram p0: block diagram]
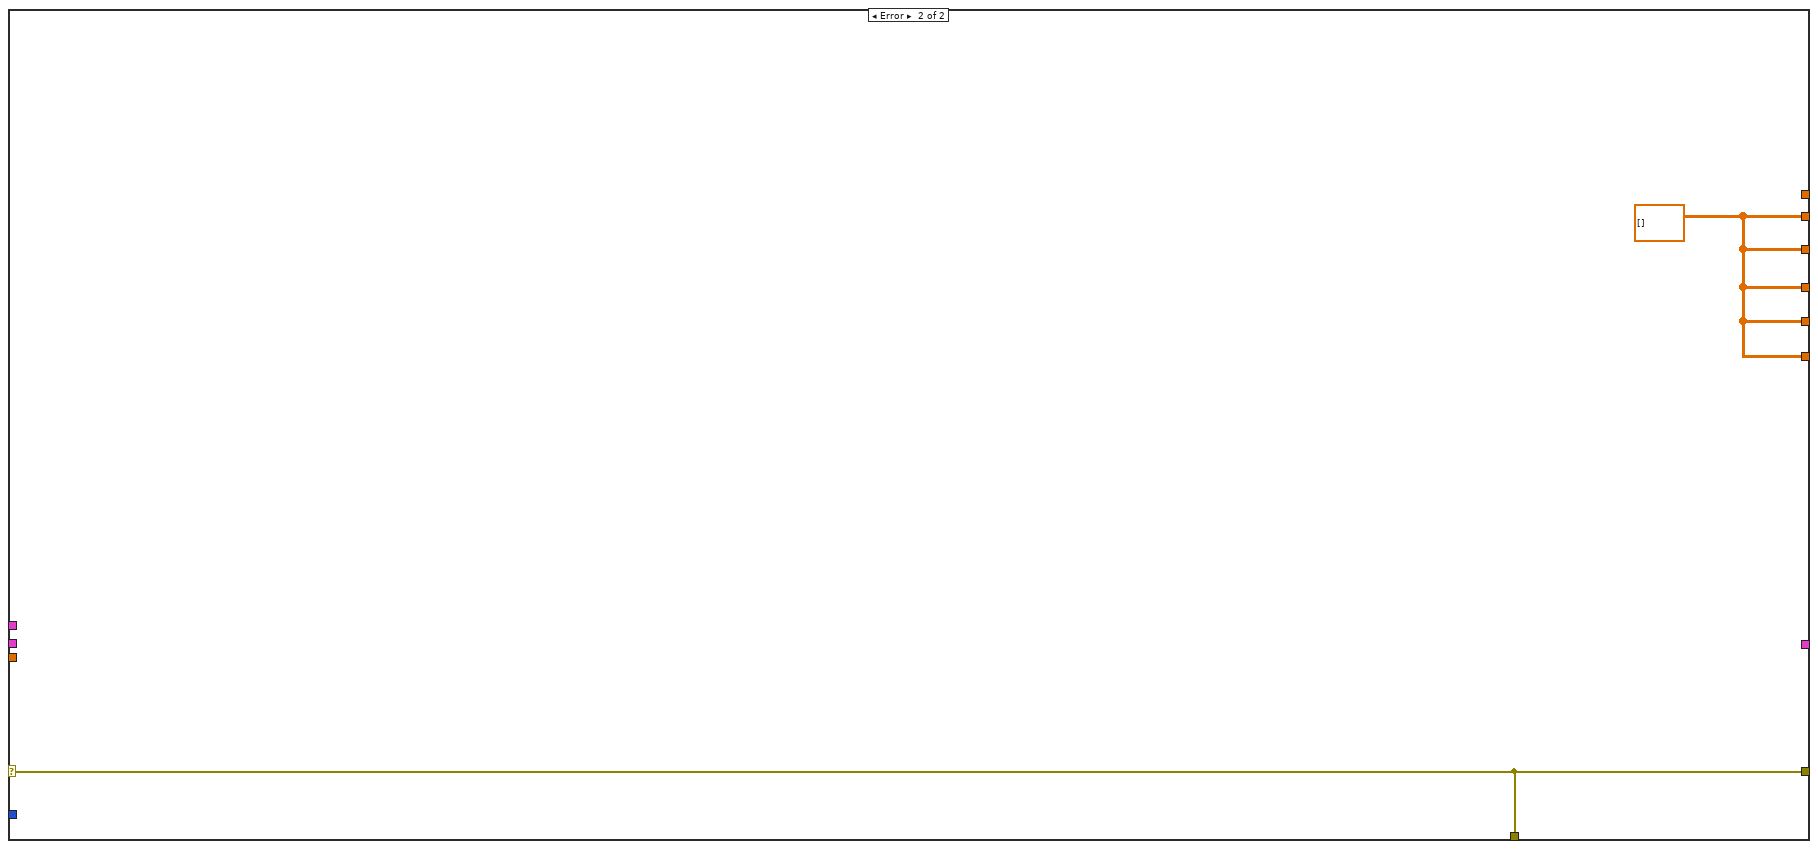
[diagram p4: hidden frame]
diagram:
  # "Note\nscanVariables contains (in sequence)\n - AOL mode \n- Wavelength\n- Centre frequency \n- Field of view\n- Frame size \n- Dwell time\n- Axial scanning\n- Zoom [array]"
  # "Note\nThe Matlab Clear All and Close All command are now run outside this VI to speed up the code, inside the \"Matlab clear and close all.vi\", which takes 12ms to execute."
  n1 = case shown="True" "Stantalone {F} ?" {
    tunnel: "error in" -> [w20 w22]
    tunnel: [w20 w21] -> w7
    frame False {
    }
    frame True {
      n2 = call "Send path to matlab.vi"("error in"=w22) -> ("error out"=w21:errorcluster)  [unwired: 10 in]
    }
  }
  n3 = Tick Count (ms)() -> (millisecond timer value=w14:u32)
  n4 = case shown="No Error" w7 {
    selector: w7 -> [w39 w60]
    tunnel: [w47 w60] -> w17
    tunnel: "ROI Coordinates" -> [w53 _]
    tunnel: "AOL_Globals" -> [w33 _]
    tunnel: [w50 _] -> w11
    tunnel: [w49 _] -> w12
    tunnel: "Zoom" -> [w40 _]
    tunnel: w14 -> [_ _]
    tunnel: [w47 w60] -> w10
    tunnel: [w30 w59] -> _
    tunnel: [w29 w59] -> _
    tunnel: [w28 w59] -> _
    tunnel: [w27 w59] -> w6
    tunnel: [w26 w59] -> w2
    frame No Error {
      # "MatLab Interface"
      n5 = Unbundle By Name(w33) -> ("Variable Miniscan Pixels"=w32:u16[])
      n6 = Boolean To (0,1)(Boolean="Movement correction") -> (0, 1=w24:i16)
      n7 = To Double Precision Float(number=w24) -> (double precision float=w23:dbl)
      n8 = To Double Precision Float(number=w32) -> (double precision float=w31:dbl[])
      n9 = call "bundleScanParameters.vi"("error in (no error)"=w39, "Zoom"=w40, "xyzNormalizedCoordinates"=w53, "AOL_Globals"=w33) -> ("error out"=w38:errorcluster, "xyzImageStopNormalised"=w51:dbl[][], "xyzImageStartNormalised"=w52:dbl[][], "scanVariables"=w49:dbl[][], "XYZ Array size"=→"XYZ Array size":i32[], "Number of Miniscans"=w36:u16, "Use Variable Length"=w37:bool)  [unwired: 1 in]
      n10 = Unbundle By Name(w33) -> ("Imaging Protocol"=w34:T5)
      n11 = script code="[ scanVariables,xyzNormalised] = variableConstruct( scanVariables,xyzImageStartNormalised,xyzImageStopNormalised);\n\n%aol_params = default.aol_params(Wavelength, Objective); \n\nimaging_mode =  ImagingMode(scanVariables.aolMode);\n\n%imaging_mode = 'raster';\n\n    non_default_aa = scanVariables.acceptanceAngle ./ scanVariables.zoomFactor(1);\n    non_default_resolution = scanVariables.numberOfVoxels;\n    non_default_dwell_time = scanVariables.dwellTime;\n    non_default_Xspin_deg =  scanVariables.Xspin_deg;\n    non_default_Yspin_deg =  scanVariables.Yspin_deg;\n    non_default_Zspin_deg =  scanVariables.Zspin_deg;\n\n  \nscan_params = default.scan_params(imaging_mode,non_default_resolution,...\nnon_default_aa,non_default_dwell_time, non_default_Xspin_deg, non_default_Yspin_deg, non_default_Zspin_deg )\n[t, a, b, c, d, aa, bb, cc, delta_bz, delta_a_dz, d_4app, numvox, stime, scan_params, aol_params, xyzNormalised, timing_offsets, distortion_corr] = ...\nlabview_interface(scanVariables, xyzNormalised, aol_params, scan_params, voxelsperramp, mc)"("??"=w38, "scanVariables"=w49, "xyzImageStartNormalised"=w52, "xyzImageStopNormalised"=w51, "voxelsperramp"=w31, "mc"=w23) -> ("??"=w47:errorcluster, "t"=w27:dbl[][], "a"=w26:dbl[][], "b"=w30:dbl[][], "c"=w29:dbl[][], "d"=w28:dbl[][], "delta_bz"=w46:dbl[][], "delta_a_dz"=w45:dbl[][], "d_4app"=w44:dbl[][], "timing_offsets"=w42:dbl[][], "distortion_corr"=w43:dbl)
      "t" <- w27
      "A" <- w26
      "B" <- w30
      "C" <- w29
      "D" <- w28
      "delta_bz" <- w46
      "delta_a_dz" <- w45
      "d_4app" <- w44
      "Distortion corr" <- w43
      "Timing_offsets" <- w42
      n12 = case shown="\"Functional Acquisition\"" w34 {
        tunnel: w37 -> [_ w58]
        tunnel: w36 -> [_ w57]
        tunnel: w26 -> [_ w56]
        tunnel: w31 -> [_ w54]
        frame Default {
        }
        frame "Functional Acquisition" {
          n13 = Array Size(array=w56) -> (size(s)=→"Chirp Array size":i32[])
          "Use Variable Length" <- w58
          "Number of Miniscans" <- w57
          "Pixels per miniscan" <- w54
        }
      }
      n14 = Index Array(array=w42) -> (element=w41:dbl[])  [unwired: 2 in]
      "timings_offsets" <- w41
      n15 = Bundle By Name(cluster=T2 {"M "=0.0, "Tramp"=[], "A"=[], "B"=[], "C"=[], "D"=[], "delta_bz"=[], "delta_a_dz"=[], "d_4app"=[], "timings_offsets"=[], "distortion_corr"=0.0} ("Chirp Parameters"), "Tramp"=w27, "A"=w26, "B"=w30, "C"=w29, "D"=w28, "delta_bz"=w46, "delta_a_dz"=w45, "d_4app"=w44, "timings_offsets"=w41, "distortion_corr"=w43) -> (w50:T2)
    }
    frame Error {
      w59 = dbl[][] []
    }
  }
  "error out" <- w17
  "Chirp Parameters" <- w11
  "scanVariables" <- w12
  n16 = flat-sequence {
    tunnel: [w61] -> w15
    tunnel: w10 -> [_]
    frame #0 {
      n17 = Tick Count (ms)() -> (millisecond timer value=w61:u32)
    }
  }
  n18 = call "Plot record data.vi"("Array"=w6) -> ("Intensity Graph"=→"T_ramp Intensity Graph":dbl[][], "All"=→"T_ramp All":dbl[][])  [unwired: 5 in, 4 out]
  n19 = call "Plot record data.vi"("Array"=w2) -> ("Intensity Graph"=→"A Intensity Graph 2":dbl[][], "All"=→"A  All":dbl[][])  [unwired: 5 in, 4 out]
  n20 = Subtract(x=w15, y=w14) -> (x-y=→"Execution time (ms)":u32)
